vi "VS_Wait.vi"(0 "delay (s)":sgl=1.0, 2 "Info In":cluster{"Numeric":u8}) -> (1 "Reply":string, 4 "Info Out":cluster{"Numeric":u8})   [LabVIEW 2014]
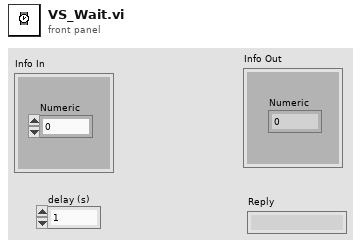
[diagram p1: front panel]
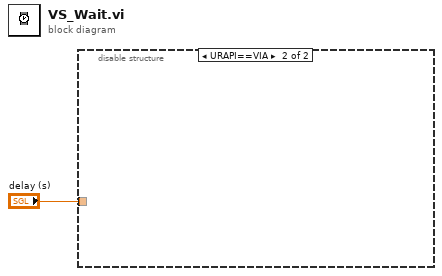
[diagram p0: block diagram]
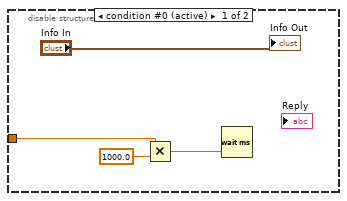
[diagram p2: hidden frame]
diagram:
  n1 = disable-structure shown="URAPI==VIA" {
    disable-tunnel: "delay (s)" -> [w4 _]
    frame condition #0 (active) {
      n2 = Multiply(x=w4, y=sgl 1000.0) -> (x*y=w2:sgl)
      n3 = Wait (ms)(milliseconds to wait=w2) -> ()  [unwired: 1 out]
      "Info Out" <- "Info In"
    }
    frame condition #1 {
    }
  }
